vi "Drive Controller.vi"(8 "error in":errorcluster) -> ()   [LabVIEW 2019]
doc: "This VI executes continuously carrying out the current operation and responding to updates or new operation requests. It will often contain the timing or control code that is difficult to place directly in TeleOp. This VI generally opens all sensors and motors and isolates the rest of the robot code from knowing implementation details of how the operations are carried out."
uses:
  <vilib>/Rock Robotics/WPI/Framework/Completion Status.ctl
  Drive Setpoints.ctl
  Drive Operations.ctl
  <vilib>/Rock Robotics/WPI/SafetyOutput/WPI_SafetyOutputConfigMenu.ctl
  <vilib>/Rock Robotics/WPI/ThirdParty/Phoenix-LabVIEW/Motor Controller/Controls/CTRE_Phoenix_MotorControl_ControlMode.ctl
  <vilib>/Rock Robotics/WPI/RobotDrive/WPI_RobotDriveOpen2MotorWithVictorSPX.vi
panel:
  in  "Interactive Values":T1
  in  "Buttons":cluster{"Execute Cmd":bool, "Abort Cmd":bool}
  out "Command Timing":cluster{"Start Time (ms)":u32, "Iterations":i32}
  out "Status":T3
  out "Setpoints":T4(graph)
  out "Current\nCmd":string
  # "Tip: The graph shows the motor setpoints. It may also be helpful to observe inputs and sensor values.\nYou may also want to display tuning or debugging controls."
  # "Interactive Command: You may fill in the settings for a command\nand schedule it with the Execute button. You can observe and abort\nany command while fine tuning the code for the controller."
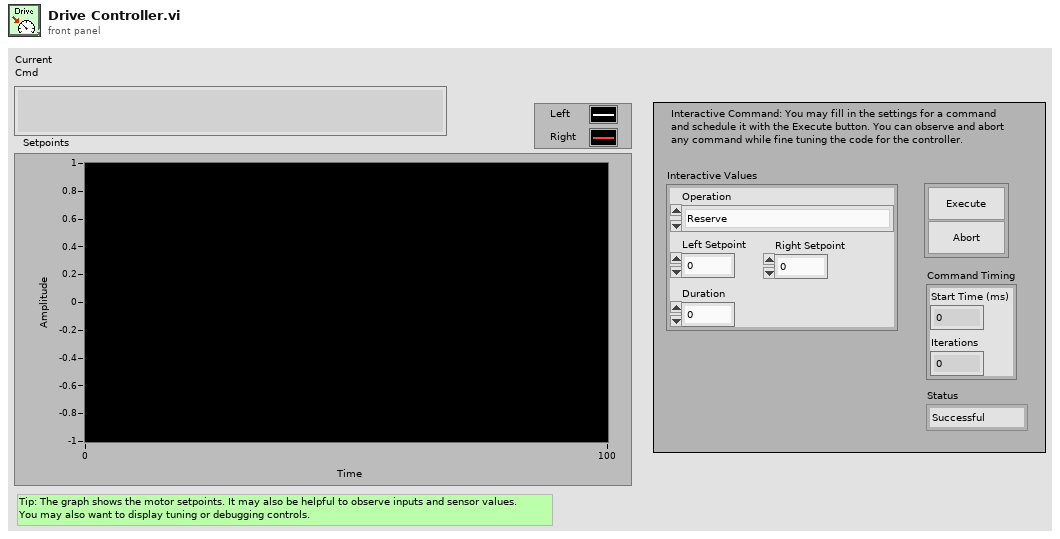
[diagram p1: front panel]
types:
  T1 = typedef "Drive Setpoints.ctl" = cluster{"Operation":T2, "Left Setpoint":dbl, "Right Setpoint":dbl, "Duration":dbl}
  T2 = typedef "Drive Operations.ctl" = enum16{"Reserve", "Read Current", "Immediate", "Drive for Time", "Drive for Distance"}
  T3 = typedef "Completion Status.ctl" = enum16{"Successful", "Aborted", "Incomplete"}
  T4 = cluster{"Left Setpoint":dbl, "Right Setpoint":dbl}
  T5 = typedef "WPI_SafetyOutputConfigMenu.ctl" = enum16{"Enable", "Disable"}
  T6 = typedef "WPI_RobotDriveDevRef.ctl" = cluster{"DevStatus":errorcluster, "Motors[]":T7[], "Square Inputs":bool, "Max Output":dbl}
  T7 = typedef "WPI_MotorControlDeviceRef.ctl" = cluster{"DeviceStatus":errorcluster, "Type":T8, "PWM":cluster{"PWM Channel":T9, "DeadBand":T10}, "CAN":cluster{"Device Number":u8, "SetOutput VI Ref":variant, "GetOutput VI Ref":variant, "Enable VI Ref":variant, "Disable VI Ref":variant, "Data":variant}, "Invert":bool, "DIO PWM":cluster{"PWM \"Enable\" Channel":T9, "DIOChannel":T11, "PWM Rate":dbl}}
  T8 = typedef "WPI_MotorControlType.ctl" = enum16{"PWM", "CAN", "DIO PWM"}
  T9 = typedef "FPGA_DIOPWMChannel.ctl" = enum8{"PWM 0", "PWM 1", "PWM 2", "PWM 3", "PWM 4", "PWM 5", "PWM 6", "PWM 7", "PWM 8", "PWM 9", "PWM MXP 0", "PWM MXP 1", "PWM MXP 2", "PWM MXP 3", "PWM MXP 4", "PWM MXP 5", "PWM MXP 6", "PWM MXP 7", "PWM MXP 8", "PWM MXP 9", "Invalid"}
  T10 = typedef "WPI_PWMDeadband.ctl" = cluster{"Name":string, "maxPositivePwm":i32, "minPositivePwm":i32, "centerPwm":i32, "maxNegativePwm":i32, "minNegativePwm":i32, "angularRange":u16}
  T11 = typedef "FPGA_DIOChannel.ctl" = enum8{"DIO 0", "DIO 1", "DIO 2", "DIO 3", "DIO 4", "DIO 5", "DIO 6", "DIO 7", "DIO 8", "DIO 9", "DIO MXP 0", "DIO MXP 1", "DIO MXP 2", "DIO MXP 3", "DIO MXP 4", "DIO MXP 5", "DIO MXP 6", "DIO MXP 7", "DIO MXP 8", "DIO MXP 9", "DIO MXP 10", "DIO MXP 11", "DIO MXP 12", "DIO MXP 13", "DIO MXP 14", "DIO MXP 15", "SPI Port CS1", "SPI Port CS2", "SPI Port CS3", "SPI Port MISO", "SPI Port MOSI", "Invalid"}
  T12 = typedef "Command Status Info.ctl" = cluster{"Name":string, "Status":T3, "notifier out":T13}
  T13 = typedef "Completion Notifier.ctl" = refnum<notifier>
  T14 = cluster{"SubSystem Data":T1, cluster{"Start Time (ms)":u32, "Iterations":i32}, cluster{"Command Info":T12, "Description":string, "Default Command":T1, "queue out":refnum<queue>, "Subsystem Name":string}}
  T15 = typedef "CTRE_Phoenix_MotorControl_ControlMode.ctl" = u16
  T16 = cluster{"SubSystem Data":T1, cluster{"Start Time (ms)":u32, "Iterations":i32}, "Default Command Arguments":cluster{"Command Info":T12, "Description":string, "Default Command":T1, "queue out":refnum<queue>, "Subsystem Name":string}}
  T17 = cluster{"Don't move motors while reserved":dbl, "Don't move motors while reserved":dbl}
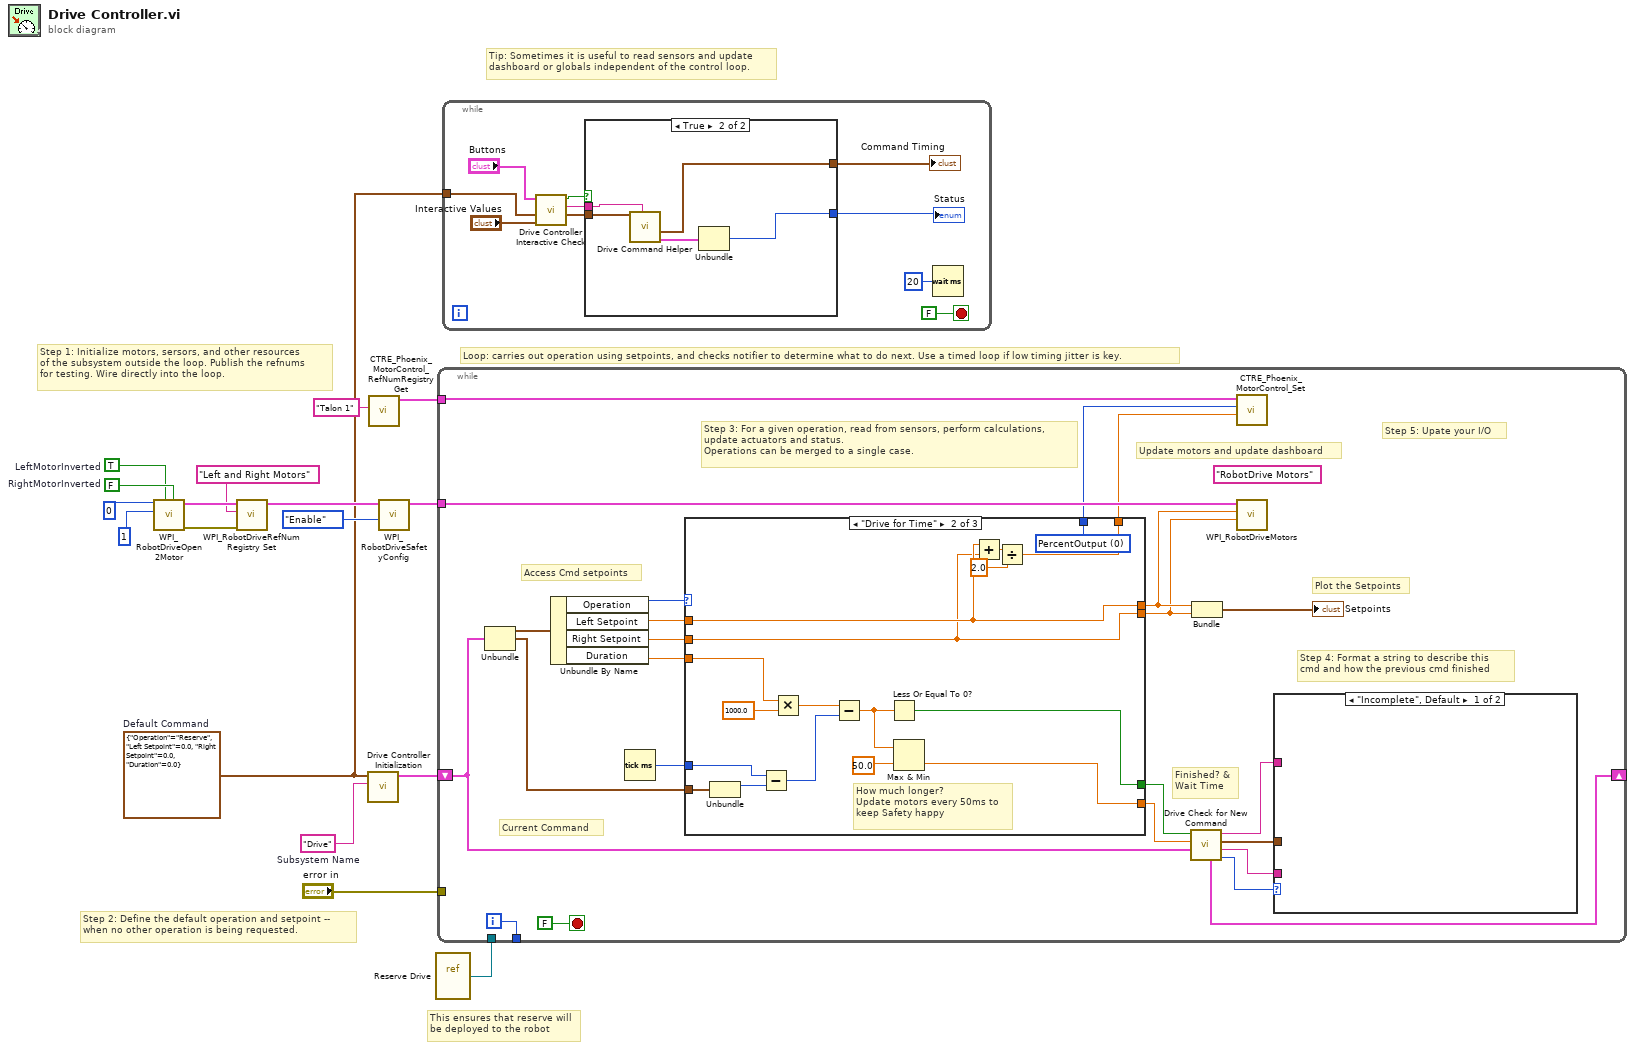
[diagram p0: block diagram]
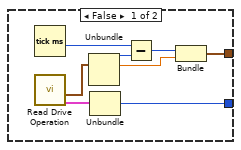
[diagram p2: hidden frame]
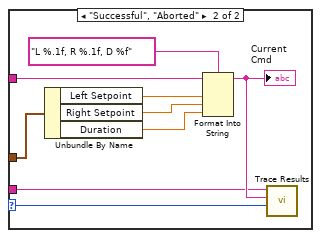
[diagram p3: hidden frame]
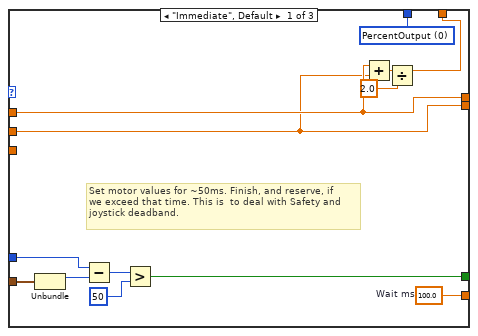
[diagram p4: hidden frame]
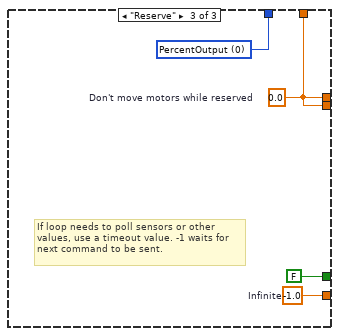
[diagram p5: hidden frame]
diagram:
  w13 = TRUE  # LeftMotorInverted
  w14 = FALSE  # RightMotorInverted
  w3 = T1 {"Operation"=enum."Reserve", "Left Setpoint"=0.0, "Right Setpoint"=0.0, "Duration"=0.0}  # Default Command
  w17 = "Drive"  # Subsystem Name
  # "This ensures that reserve will\nbe deployed to the robot"
  # "Tip: Sometimes it is useful to read sensors and update\ndashboard or globals independent of the control loop."
  # "Step 2: Define the default operation and setpoint --\nwhen no other operation is being requested."
  # "Step 1: Initialize motors, sersors, and other resources\nof the subsystem outside the loop. Publish the refnums\nfor testing. Wire directly into the loop."
  # "Loop: carries out operation using setpoints, and checks notifier to determine what to do next. Use a timed loop if low timing jitter is key."
  n1 = call-poly <vilib>:"WPI_RobotDriveOpen2Motor.vi"("Right Motor Inverted"=w14, "Left Motor Inverted"=w13, "Right Motor"=u8 1 ("Left Motor"), "Left Motor"=u8 0) -> ("error out"=w10:errorcluster, "RobotDriveDevRef"=w12:T6)  [unwired: 1 in, 5 out]
  n2 = call <vilib>:"WPI_RobotDriveRefNum Registry Set.vi"("error in (no error)"=w10, "refnum name"="Left and Right Motors", "RobotDriveDevRef"=w12) -> ("RobotDriveDevRef"=w9:T6)  [unwired: 1 in, 7 out]
  n3 = call "Drive Controller Initialization.vi"("Subsystem Name"=w17, "Default Command"=w3) -> ("Current Command"=w5:T14)  [unwired: 9 in]
  n4 = call <vilib>:"CTRE_Phoenix_MotorControl_RefNumRegistryGet.vi"("refnum name"="Talon 1") -> ("PhoenixMotorControlDevRef"=w1:T7)  [unwired: 9 in, 1 out]
  n5 = call <vilib>:"WPI_RobotDriveSafetyConfig.vi"("mode"=WPI_SafetyOutputConfigMenu."Enable", "RobotDriveDevRef"=w9) -> ("RobotDriveDevRef"=w7:T6)  [unwired: 8 in, 1 out]
  n6 = vi-ref "Reserve Drive.vi"() -> (w4:refnum<vi>)
  n7 = while {
    shift-right: [w28] -> _
    shift-left: w5 -> [w21]
    tunnel: [w40] -> _
    tunnel: w7 -> [w36]
    tunnel: "error in" -> [_]
    tunnel: w4 -> [_]
    tunnel: w1 -> [w20]
    i -> [w40]
    stop <- FALSE stop-if-true
    (unwired) "RobotDrive Motors" ("Name")
    # "Step 5: Upate your I/O"
    # "Step 4: Format a string to describe this\ncmd and how the previous cmd finished"
    # "Current Command"
    # "Update motors and update dashboard"
    # "Plot the Setpoints"
    # "Access Cmd setpoints"
    # "Finished? &\nWait Time"
    # "Step 3: For a given operation, read from sensors, perform calculations,\nupdate actuators and status.\nOperations can be merged to a single case."
    n8 = Unbundle(w21) -> ("SubSystem Data"=w35:T1, w22:cluster{"Start Time (ms)":u32, "Iterations":i32})  [unwired: 1 out]
    n9 = Unbundle By Name(w35) -> ("Operation"=w34:T2, "Left Setpoint"=w33:dbl, "Right Setpoint"=w32:dbl, "Duration"=w31:dbl)
    n10 = Tick Count (ms)() -> (millisecond timer value=w30:u32)
    n11 = case shown="\"Drive for Time\"" w34 {
      tunnel: [w63 w70 w84] -> w27
      tunnel: [w58 w75 FALSE ("ignore previous (F)")] -> w26
      tunnel: w22 -> [w57 w77 _]
      tunnel: [w55 w67 w82] -> w38
      tunnel: [w54 w66 w82] -> w37
      tunnel: w33 -> [w55 w67 _]
      tunnel: w32 -> [w54 w66 _]
      tunnel: w31 -> [_ w74 _]
      tunnel: w30 -> [w59 w73 _]
      tunnel: [w52 w65 w82] -> w19
      tunnel: [w56 w64 w81] -> w18
      frame "Immediate", Default {
        w56 = T15 0 items=["PercentOutput"=0, "Position"=1, "Velocity"=2, "Current"=3, "Follower"=5, "MotionProfile"=6, "MotionMagic"=7, "MotionProfileArc"=10, "Disabled"=15] ("Control Mode")
        w63 = 100.0  # Wait ms
        # "Set motor values for ~50ms. Finish, and reserve, if\nwe exceed that time. This is  to deal with Safety and\njoystick deadband."
        n12 = Unbundle(w57) -> ("Start Time (ms)"=w60:u32)  [unwired: 1 out]
        n13 = Subtract(x=w59, y=w60) -> (x-y=w61:u32)
        n14 = Greater?(x=w61, y=u8 50 ("Left Motor")) -> (0:w58:bool)
        n15 = Add(x=w55, y=w54) -> (x+y=w53:dbl)
        n16 = Divide(x=w53, y=2.0) -> (x/y=w52:dbl)
      }
      frame "Drive for Time" {
        w64 = T15 0 items=["PercentOutput"=0, "Position"=1, "Velocity"=2, "Current"=3, "Follower"=5, "MotionProfile"=6, "MotionMagic"=7, "MotionProfileArc"=10, "Disabled"=15] ("Control Mode")
        # "How much longer?\nUpdate motors every 50ms to\nkeep Safety happy"
        n17 = Unbundle(w77) -> ("Start Time (ms)"=w76:u32)  [unwired: 1 out]
        n18 = Subtract(x=w73, y=w76) -> (x-y=w80:u32)
        n19 = Multiply(x=w74, y=1000.0) -> (x*y=w79:dbl)
        n20 = Subtract(x=w79, y=w80) -> (x-y=w72:dbl)
        n21 = Less Or Equal To 0?(x=w72) -> (x <= 0?=w75:bool)
        n22 = Max & Min(x=w72, y=50.0) -> (min(x,y)=w70:dbl)  [unwired: 1 out]
        n23 = Add(x=w67, y=w66) -> (x+y=w69:dbl)
        n24 = Divide(x=w69, y=2.0) -> (x/y=w65:dbl)
      }
      frame "Reserve" {
        w81 = T15 0 items=["PercentOutput"=0, "Position"=1, "Velocity"=2, "Current"=3, "Follower"=5, "MotionProfile"=6, "MotionMagic"=7, "MotionProfileArc"=10, "Disabled"=15] ("Control Mode")
        w82 = 0.0  # Don't move motors while reserved
        w84 = -1.0  # Infinite
        # "If loop needs to poll sensors or other\nvalues, use a timeout value. -1 waits for\nnext command to be sent."
      }
    }
    n25 = call "Drive Check for New Command.vi"("input cluster"=w21, "Wait time (ms)"=w27, "Finished?"=w26) -> ("Completion"=w29:T3, "Subsystem Name"=w23:string, "Current Command"=w24:T1, "Initial Trace String"=w25:string, "Next Command"=w28:T16)  [unwired: 4 in]
    n26 = Bundle("Don't move motors while reserved"=w38, "Don't move motors while reserved"=w37) -> (→"Setpoints":T17)  [unwired: 1 in]
    n27 = call <vilib>:"CTRE_Phoenix_MotorControl_Set.vi"("Output"=w19, "Control Mode"=w18, "PhoenixMotorControlDevRef"=w20) -> ()  [unwired: 7 in, 2 out]
    n28 = call <vilib>:"WPI_RobotDriveMotors.vi"("RightSpeed"=w37, "LeftSpeed"=w38, "RobotDriveDevRef"=w36) -> ()  [unwired: 1 in, 8 out]
    n29 = case shown="\"Incomplete\", Default" w29 {
      selector: w29 -> [_ w50]
      tunnel: w25 -> [_ w45]
      tunnel: w24 -> [_ w46]
      tunnel: w23 -> [_ w42]
      frame "Incomplete", Default {
        # "Continuing current command"
      }
      frame "Successful", "Aborted" {
        # "Report and setup for next command"
        n30 = Unbundle By Name(w46) -> ("Left Setpoint"=w48:dbl, "Right Setpoint"=w49:dbl, "Duration"=w43:dbl)
        n31 = Format Into String(format string="L %.1f, R %.1f, D %f", initial string=w45, w48, w49, w43) -> (resulting string=w44:string)  [unwired: 1 in, 1 out]
        "Current\nCmd" <- w44
        n32 = call <vilib>:"Trace Results.vi"("Status of previous command"=w50, "Description"=w44, "Subsystem"=w42) -> ()  [unwired: 9 in]
      }
    }
  }
  n33 = while {
    tunnel: w3 -> [w86]
    stop <- FALSE stop-if-true
    n34 = call "Drive Controller Interactive Check.vi"("Interactive Command In"="Interactive Values", "Default Command"=w86, "Buttons"="Buttons") -> ("Interactive Command Out"=w88:T1, "Trace String"=w89:string, "Schedule"=w90:bool)  [unwired: 6 in]
    n35 = case shown="True" w90 {
      tunnel: [w99 w107] -> w91
      tunnel: [w98 w103] -> w92
      tunnel: w89 -> [_ w105]
      tunnel: w88 -> [_ w104]
      frame False {
        n36 = Tick Count (ms)() -> (millisecond timer value=w102:u32)
        n37 = call "Read Drive Operation.vi"() -> ("Command Info"=w96:T12, "SubSystem Data"=w95:T1)  [unwired: 9 in, 1 out]
        n38 = Unbundle(w95) -> ("Operation"=w100:T2, "Left Setpoint"=w97:dbl)  [unwired: 2 out]
        n39 = Unbundle(w96) -> ("Status"=w99:T3)  [unwired: 2 out]
        n40 = Subtract(x=w102, y=w100) -> (x-y=w101:u32)
        n41 = Bundle(w101, "Left Setpoint"=w97) -> (w98:cluster{u32, "Left Setpoint":dbl})  [unwired: 1 in]
      }
      frame True {
        n42 = call "Drive Command Helper.vi"("Description"=w105, "SubSystem Data"=w104) -> ("Command Info Out"=w106:T12, "Command Timing"=w103:cluster{"Start Time (ms)":u32, "Iterations":i32})  [unwired: 7 in, 1 out]
        n43 = Unbundle(w106) -> ("Status"=w107:T3)  [unwired: 2 out]
      }
    }
    "Status" <- w91
    "Command Timing" <- w92
    n44 = Wait (ms)(milliseconds to wait=u32 20) -> ()  [unwired: 1 out]
  }
